vi "Serialize Cluster.vi"(8 "error in (no error)":errorcluster, 11 "Serializer in":refnum<class "Serializer.lvclass">) -> (0 "error out":errorcluster, 3 "Serializer out":refnum<class "Serializer.lvclass">)   [LabVIEW 2014, in "Serializer.lvclass"]
uses:
  Serializer.lvclass
panel:
  out "ClusterIn":variant
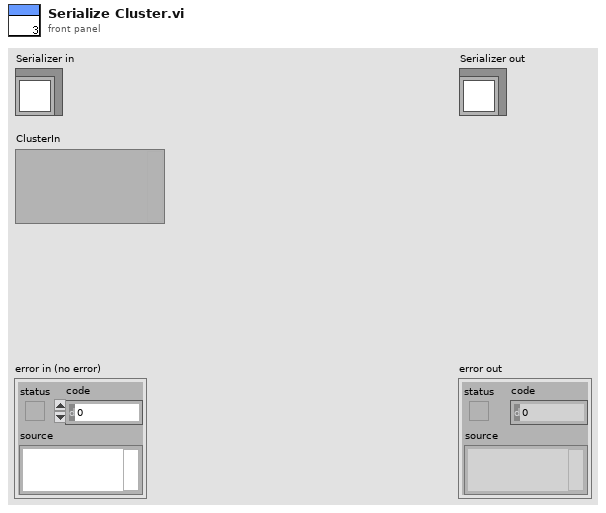
[diagram p1: front panel]
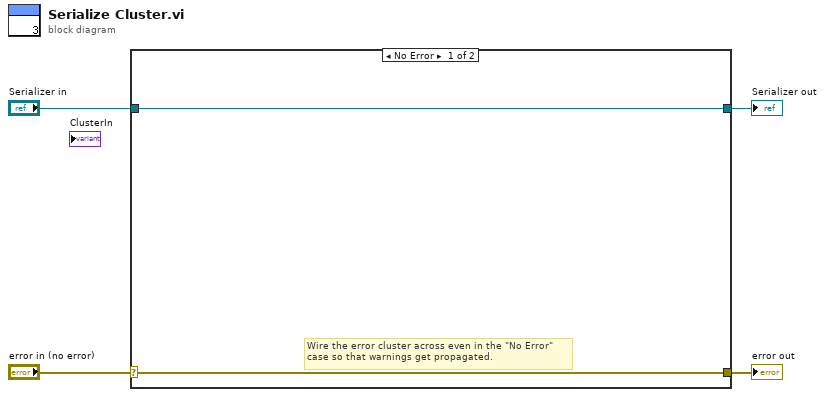
[diagram p0: block diagram]
diagram:
  n1 = case shown="No Error" "error in (no error)" {
    selector: "error in (no error)" -> [w5 w8]
    tunnel: [w5 w8] -> w3
    tunnel: [w6 w7] -> w1
    tunnel: "Serializer in" -> [w6 w7]
    frame No Error {
      # "Wire the error cluster across even in the \"No Error\"\ncase so that warnings get propagated."
    }
    frame Error {
    }
  }
  "error out" <- w3
  "Serializer out" <- w1
